vi "ExFilterWheel.vi"() -> ()   [LabVIEW 2010]
panel:
  out "User Name":string
  out "Serial Number":string
  out "Model Name":string
  out "Model Number":u32
  in  "?":bool
  out "Number of Filter Wheels":i16
  in  "?":bool
  out "Filter Wheel Open":bool
  out "Number Of Filters":i16=1 min=1 step=1
  in  "?":bool
  in  "?":bool
  out "Filter":i16=1 min=1 step=1
  in  "?":bool
  in  "?":bool
  in  "?":bool
  in  "Filter":i16=1 min=1 max=100 step=1
  out "error out":errorcluster
  in  "error in":errorcluster
  # "ExFilterWheel.vi\n(Normal filter wheel via USB/COM port)\nThis example shows how access a filter wheel via a USB/COM port.\nNot all commands may be available for all filter wheels.\nNOTE: The properly configured filter wheel .ini file must be\npresent in the LabVIEW folder for filter wheel operation."
  # "This is the number of filter\nwheels setup in the .ini file."
  # "The number of filters is set in the .ini file"
  # "Note: Model Number,\nModel Name and\nSerial Number are\nobtained from the filter\nwheel.  If it does not\ncarry this information,\nthese values will be 0\nor blank.  The User\nName is taken from\nthe .ini file."
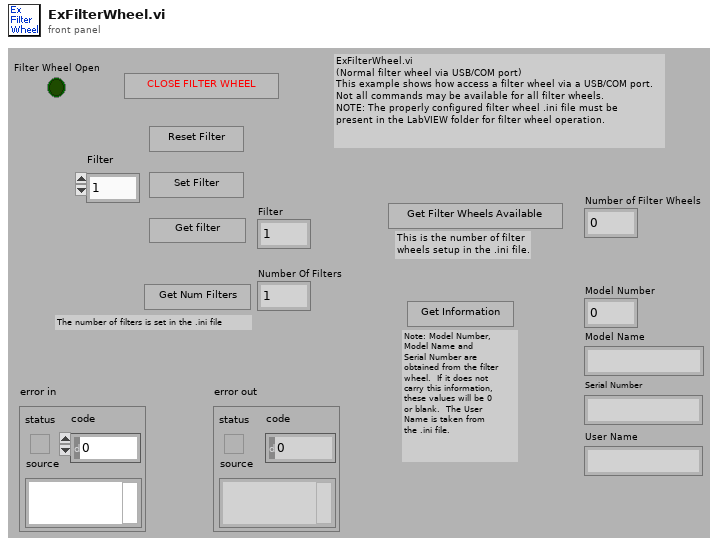
[diagram p1: front panel]
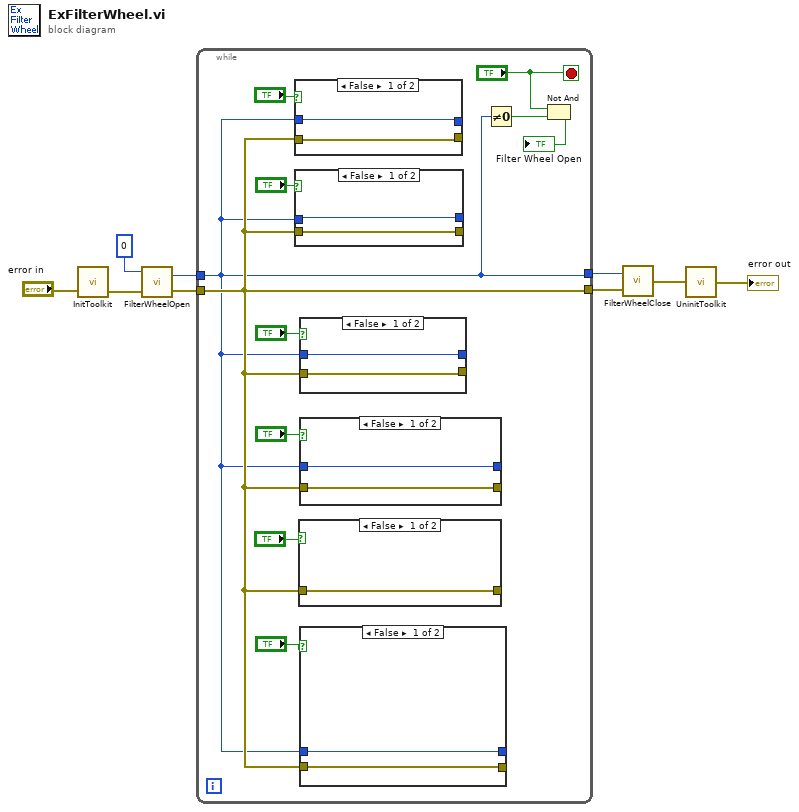
[diagram p0: block diagram]
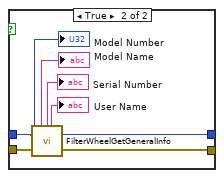
[diagram p2: hidden frame]
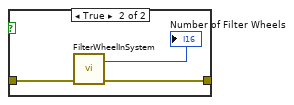
[diagram p3: hidden frame]
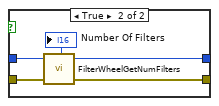
[diagram p4: hidden frame]
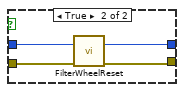
[diagram p5: hidden frame]
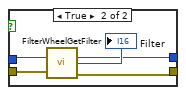
[diagram p6: hidden frame]
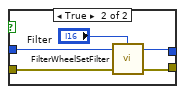
[diagram p7: hidden frame]
diagram:
  n1 = call <userlib>:"InitToolkit.vi"("error in"="error in") -> ("error out"=w8:errorcluster)
  n2 = call <userlib>:"FilterWheelOpen.vi"("error in"=w8, "Filter Wheel ID"=0) -> ("error out"=w4:errorcluster, "Filter Wheel Handlle"=w1:u32)  [unwired: 1 in]
  n3 = while {
    tunnel: w1 -> [w10]
    tunnel: w4 -> [w11]
    tunnel: [w10] -> w3
    tunnel: [w11] -> w2
    stop <- "?" stop-if-true
    n4 = case shown="False" "?" {
      tunnel: [w55 w61] -> _
      tunnel: [w56 w60] -> _
      tunnel: w10 -> [w56 w59]
      tunnel: w11 -> [w55 w58]
      frame False {
      }
      frame True {
        n5 = call <userlib>:"FilterWheelSetFilter.vi"("error in"=w58, "Filter"="Filter", "Filter Wheel Handle"=w59) -> ("error out"=w61:errorcluster, "Filter Wheel Handle"=w60:u32)  [unwired: 1 in]
      }
    }
    n6 = case shown="False" "?" {
      tunnel: w10 -> [w49 w54]
      tunnel: w11 -> [w48 w53]
      tunnel: [w48 w52] -> _
      tunnel: [w49 w50] -> _
      frame False {
      }
      frame True {
        n7 = call <userlib>:"FilterWheelGetFilter.vi"("error in"=w53, "Filter Wheel Handle"=w54) -> ("error out"=w52:errorcluster, "Filter Number"=→"Filter":i16, "Filter Wheel Handle"=w50:u32)  [unwired: 1 in]
      }
    }
    n8 = case shown="False" "?" {
      tunnel: w11 -> [w31 w34]
      tunnel: [w31 w33] -> _
      frame False {
      }
      frame True {
        n9 = call <userlib>:"FilterWheelInSystem.vi"("error in"=w34) -> ("Number of Filter Wheels"=→"Number of Filter Wheels":i32, "error out"=w33:errorcluster)
      }
    }
    n10 = case shown="False" "?" {
      tunnel: w11 -> [w42 w45]
      tunnel: w10 -> [w43 w47]
      tunnel: [w43 w46] -> _
      tunnel: [w42 w44] -> _
      frame False {
      }
      frame True {
        n11 = call <userlib>:"FilterWheelReset.vi"("error in"=w45, "Filter Wheel Handle"=w47) -> ("error out"=w44:errorcluster, "Filter Wheel Handle"=w46:u32)  [unwired: 1 in]
      }
    }
    n12 = case shown="False" "?" {
      tunnel: w10 -> [w36 w40]
      tunnel: [w36 w39] -> _
      tunnel: w11 -> [w35 w38]
      tunnel: [w35 w37] -> _
      frame False {
      }
      frame True {
        n13 = call <userlib>:"FilterWheelGetNumFilters.vi"("error in"=w38, "Filter Wheel Handle"=w40) -> ("error out"=w37:errorcluster, "Number of Filters"=→"Number Of Filters":i16, "Filter Wheel Handle"=w39:u32)  [unwired: 1 in]
      }
    }
    n14 = case shown="False" "?" {
      tunnel: w11 -> [w21 w25]
      tunnel: w10 -> [w22 w26]
      tunnel: [w21 w24] -> _
      tunnel: [w22 w23] -> _
      frame False {
      }
      frame True {
        n15 = call <userlib>:"FilterWheelGetGeneralInfo.vi"("Filter Wheel Handle"=w26, "error in"=w25) -> ("Model Number"=→"Model Number":u32, "User Name"=→"User Name":string, "Filter Wheel Handle"=w23:u32, "ModelName"=→"Model Name":string, "Serial Number"=→"Serial Number":string, "error out"=w24:errorcluster)
      }
    }
    n16 = Not Equal To 0?(x=w10) -> (x != 0?=w16:bool)
    n17 = Not And(1:w16, 2:"?") -> (0:→"Filter Wheel Open":bool)
  }
  n18 = call <userlib>:"FilterWheelClose.vi"("error in"=w2, "Filter Wheel Handle"=w3) -> ("error out"=w5:errorcluster)
  n19 = call <userlib>:"UninitToolkit.vi"("error in"=w5) -> ("error out"=→"error out":errorcluster)
